vi "wip.vi"   [LabVIEW 2021]
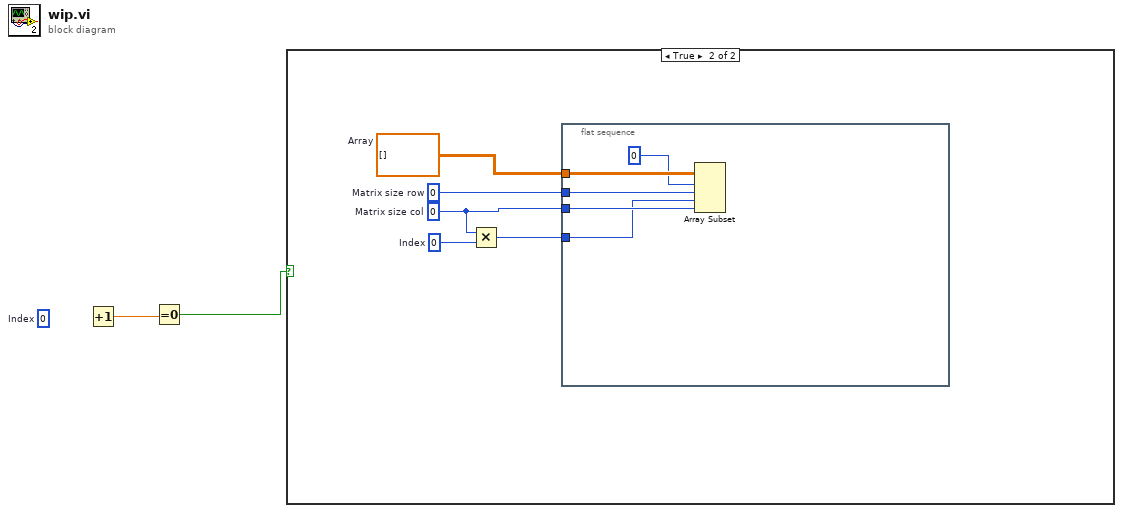
[diagram p0: block diagram]
diagram:
  (unwired) 0  # Index
  n1 = Increment() -> (x+1=w2:dbl)  [unwired: 1 in]
  n2 = Equal To 0?(x=w2) -> (x = 0?=w1:bool)
  n3 = case shown="True" w1 {
    frame False {
    }
    frame True {
      w6 = 0  # Matrix size row
      w7 = dbl[][] []  # Array
      w5 = 0  # Matrix size col
      w4 = 0  # Index
      n4 = Multiply(x=w5, y=w4) -> (x*y=w3:i32)
      n5 = flat-sequence {
        tunnel: w7 -> [w12]
        tunnel: w5 -> [w9]
        tunnel: w6 -> [w11]
        tunnel: w3 -> [w8]
        frame #0 {
          n6 = Array Subset(array=w12, index (row)=0 ("index"), length (row)=w11, index (col)=w8, length (col)=w9) -> ()  [unwired: 1 out]
        }
      }
    }
  }
